vi "AutoFocus Data.vi"() -> (0 "AutoFocus Data":T1={"Configuration"={"Matching Criteria"={"Minimum Score"=700.0, "Color Score Weight"=700.0, "Minimum Contrast"=50, "Match Mode"=0, "Match Feature Mode"=0, "Subpixel Accuracy"=TRUE, "Color Sensitivity"=1, "Search Strategy"=1}, "Z Scan Parameters"={"Z Range"=1380.0, "Resolution"=5000.0, "Initial Direction"=enum."Up", "Focus Threshold"=0.1, "Ascent Constant"=0.1}, "Displacement"=0.0, "Transformation Matrix"=[]}, "Refnums"={"Instrument Status"=refnum, "Matching Criteria"=refnum, "Z Scan Parameters"=refnum, "Distance"=refnum, "Transformation Matrix"=refnum, "Match and Edge"={"Image"=refnum, "Target"=refnum, "Edge"=refnum, "Target Data"=refnum}, "Matching Curves"=refnum, "Tracking"=refnum, "Focus"=refnum, "Find Focus"=refnum, "Set Target"=refnum, "Link Stage & Camera"=refnum, "Align"=refnum}, "Initialize"={"Update Refnums"=FALSE, "Allocate Image Memory"=FALSE, "Set Match Criteria"=FALSE, "Link Stage & Camera"=FALSE, "Set Target"=FALSE, "Find Target"=FALSE}} {"Configuration"."Displacement" scale=1.0..1000.0; "Configuration"."Z Scan Parameters"."Focus Threshold" min=0.0 max=1000.0 step=1.0 format="%#_2f"; "Configuration"."Z Scan Parameters"."Ascent Constant" min=0.0 max=1000.0 step=1.0 format="%#_2f"; "Configuration"."Z Scan Parameters"."Resolution" min=0.0 max=1.0 step=0.01 format="%_2g"; "Configuration"."Z Scan Parameters"."Z Range" format="%_3g"; "Configuration"."Matching Criteria"."Match Mode" items=["Shift Invariant", "Rotation Invariant"]; "Configuration"."Matching Criteria"."Match Feature Mode" items=["Color and Shape", "Color", "Shape"]; "Configuration"."Matching Criteria"."Color Sensitivity" items=["Low Sensitivity", "Medium Sensitivity", "High Sensitivity"]; "Configuration"."Matching Criteria"."Search Strategy" items=["Conservative", "Balance", "Aggressive", "Very Aggressive"]})   [LabVIEW 2014]
uses:
  AutoFocus Data.ctl
  AutoFocus Config.ctl
  ZScan.ctl
  <vilib>/Analysis/Matrix/Datatypes/RealMatrix.ctl
  AutoFocus Refnums.ctl
  support/Instrument Status.ctl
  Target Refnums.ctl
  AutoFocus Initialize.ctl
  <vilib>/Analysis/Matrix/NI_Matrix.lvlib
panel:
  # "LICENSED MATERIALS – PROPERTY OF IBM\nCopyright IBM Corp. 2016,\nALL RIGHTS RESERVED"
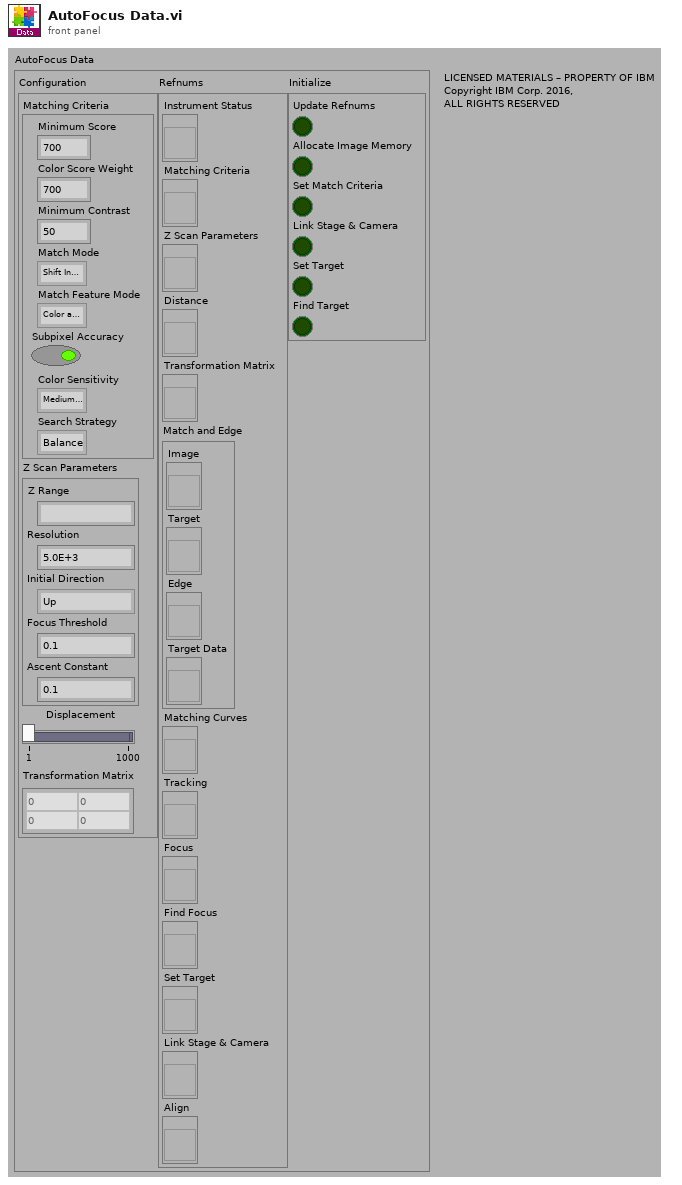
[diagram p1: front panel]
types:
  T1 = typedef "AutoFocus Data.ctl" = cluster{"Configuration":T2, "Refnums":T5, "Initialize":T7}
  T2 = typedef "AutoFocus Config.ctl" = cluster{"Matching Criteria":cluster{"Minimum Score":sgl, "Color Score Weight":sgl, "Minimum Contrast":i32, "Match Mode":u32, "Match Feature Mode":u32, "Subpixel Accuracy":bool, "Color Sensitivity":u32, "Search Strategy":u32}, "Z Scan Parameters":T3, "Displacement":dbl, "Transformation Matrix":T4}
  T3 = typedef "ZScan.ctl" = cluster{"Z Range":ext, "Resolution":dbl, "Initial Direction":enum16{"Up", "Down"}, "Focus Threshold":dbl, "Ascent Constant":dbl}
  T4 = typedef "NI_Matrix.lvlib/RealMatrix.ctl" = dbl[][]
  T5 = typedef "AutoFocus Refnums.ctl" = cluster{"Instrument Status":refnum<vi>, "Matching Criteria":refnum<vi>, "Z Scan Parameters":refnum<vi>, "Distance":refnum<vi>, "Transformation Matrix":refnum<vi>, "Match and Edge":T6, "Matching Curves":refnum<vi>, "Tracking":refnum<vi>, "Focus":refnum<vi>, "Find Focus":refnum<vi>, "Set Target":refnum<vi>, "Link Stage & Camera":refnum<vi>, "Align":refnum<vi>}
  T6 = typedef "Target Refnums.ctl" = cluster{"Image":refnum<vi>, "Target":refnum<vi>, "Edge":refnum<vi>, "Target Data":refnum<vi>}
  T7 = typedef "AutoFocus Initialize.ctl" = cluster{"Update Refnums":bool, "Allocate Image Memory":bool, "Set Match Criteria":bool, "Link Stage & Camera":bool, "Set Target":bool, "Find Target":bool}
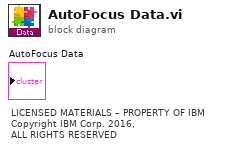
[diagram p0: block diagram]
diagram:
  # "LICENSED MATERIALS – PROPERTY OF IBM\nCopyright IBM Corp. 2016,\nALL RIGHTS RESERVED"
